vi "F Dwf Digital Out Output Get.vi"(8 "error in (no error)":errorcluster, 9 "pv":i32, 10 "idxChannel":i32, 11 "hdwf":i32) -> (0 "error out":errorcluster, 1 "pv out":i32, 3 "function return":i32)   [LabVIEW 2019, in "Olasdwf.lvlib"]
doc: "DWFAPI int FDwfDigitalOutOutputGet(HDWF hdwf, int idxChannel, DwfDigitalOutOutput *pv);"
uses:
  Olasdwf.lvlib
  Windows/System32/dwf.dll
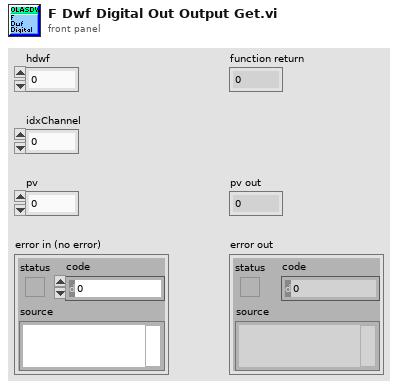
[diagram p1: front panel]
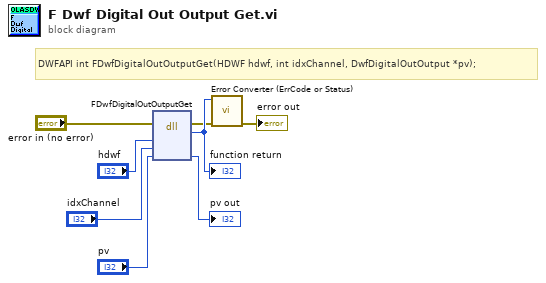
[diagram p0: block diagram]
diagram:
  # "DWFAPI int FDwfDigitalOutOutputGet(HDWF hdwf, int idxChannel, DwfDigitalOutOutput *pv);"
  n1 = dll-call lib="C:/Windows/System32/dwf.*" fn="FDwfDigitalOutOutputGet"(error in="error in (no error)", "hdwf"="hdwf", "idxChannel"="idxChannel", "pv"="pv") -> (error out=w2:errorcluster, w8:i32, "pv"=→"pv out":i32)  [unwired: 4 in, 1 out]
  "function return" <- w8
  n2 = call "Error Converter (ErrCode or Status).vi"("error in (no error)"=w2, "error code"=w8) -> ("error out"=→"error out":errorcluster)  [unwired: 9 in]
